vi "Replication and Deployment Utility.vi"() -> ()   [LabVIEW 2020]
uses:
  subVIs/TypeDefs/rad_State Data.ctl
  subVIs/Targets/TypeDefs/rad_Targets Settings.ctl
  subVIs/Targets/TypeDefs/rad_Target Information.ctl
  subVIs/Targets/TypeDefs/rad_Target Network Settings.ctl
  subVIs/App Images/TypeDefs/rad_App Images Settings.ctl
  subVIs/App Images/TypeDefs/rad_AppImage Information.ctl
  subVIs/App Images/TypeDefs/rad_Application Image Properties.ctl
  subVIs/App Images/TypeDefs/rad_FPGA Properties.ctl
  subVIs/App Images/TypeDefs/rad_FPGA Flash Properties.ctl
  subVIs/Targets/TypeDefs/rad_Discovery Settings.ctl
  subVIs/Util/Controls/Exit Button.ctl
  subVIs/Util/Controls/Retrieve Button.ctl
  subVIs/Util/Controls/Refresh Button.ctl
  subVIs/Util/Controls/Configure Button.ctl
  subVIs/Util/Controls/Deploy Button.ctl
  subVIs/Util/Controls/Select All Button.ctl
  subVIs/Util/Controls/Add Target Button.ctl
  subVIs/Util/Controls/Compare Button.ctl
  subVIs/Util/FP Control/FP Control Functions.ctl
  <vilib>/Utility/miscctls.llb/LVRowAndColumnUnsignedTypeDef.ctl
  subVIs/RT Image Compare/TypeDefs/rad_Comparison Modes.ctl
  <vilib>/nisyscfg/Close (System).vi
  subVIs/rad_Globals.vi
  <vilib>/nisyscfg/nisyscfg.lvlib
  <resource>/objmgr/nisysapi.rc
panel:
  in  "Targets Settings":bool
  in  "Refresh Targets":T1
  in  "Target List":i32[](listbox)=[0]
  in  "Add Target":T2
  in  "Select All":T3
  in  "Configure Targets":T4
  in  "Compare":T5
  in  "Deploy":T6
  in  "Retrieve":T7
  in  "State":T8 {"Targets Information"."Primary NIC"."IP Address Request Mode" items=["Static"=1, "DHCP/Link-Local"=2, "Link-Local Only"=4, "DHCP Only"=8]}
  in  "App Images Settings":bool
  in  "Refresh Apps":T1
  in  "Exit":T18
  in  "App Images List":i32(listbox)=6
  in  "Configure App":T4
  # "Deployment Targets"
  # "Application Images"
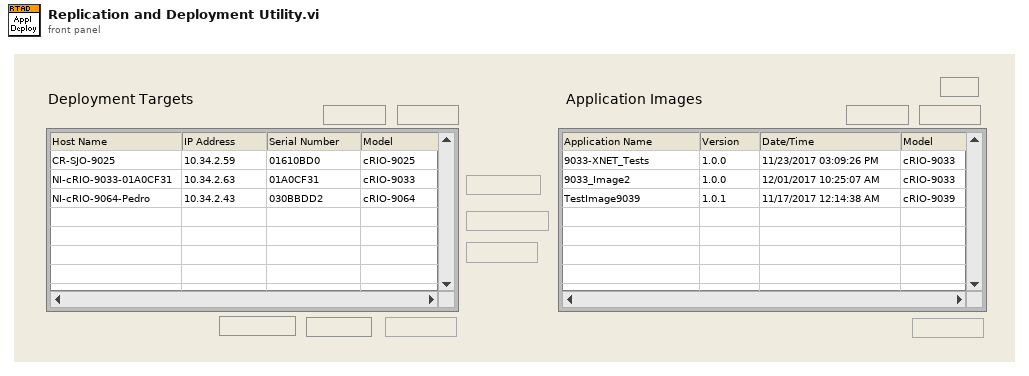
[diagram p1: front panel]
types:
  T1 = typedef "Refresh Button.ctl" = bool
  T2 = typedef "Add Target Button.ctl" = bool
  T3 = typedef "Select All Button.ctl" = bool
  T4 = typedef "Configure Button.ctl" = bool
  T5 = typedef "Compare Button.ctl" = bool
  T6 = typedef "Deploy Button.ctl" = bool
  T7 = typedef "Retrieve Button.ctl" = bool
  T8 = typedef "rad_State Data.ctl" = cluster{"Targets Settings":T9, "Targets Information":T10[], "App Images Settings":T12, "App Images Information":T13[], "Filtered Targets":i32[], "AppMode":string, "Configuration File Path":path, "Permissions":cluster{"Retrieve AppImgs":bool}, "User Added Targets":string[], "Discovery":T17}
  T9 = typedef "rad_Targets Settings.ctl" = cluster{"Target Types":string[], "Reduce Discovery Timeout":bool}
  T10 = typedef "rad_Target Information.ctl" = cluster{"Hostname":string, "Serial number":string, "Product name":string, "Product code":i32, "System status":string, "Credential type":enum16{"None/Unlocked", "FTP Password", "NIAuth Credentials"}, "User added?":bool, "Primary NIC":T11}
  T11 = typedef "rad_Target Network Settings.ctl" = cluster{"MAC address":string, "IP Address Request Mode":i32, "IP address":string, "Subnet mask":string, "Gateway":string, "DNS server":string}
  T12 = typedef "rad_App Images Settings.ctl" = cluster{"App Images Folder":path, "App Images Temp Folder":path, "CurrentVersion":string}
  T13 = typedef "rad_AppImage Information.ctl" = cluster{"AppImage Properties":T14, "AppImage Path":path}
  T14 = typedef "rad_Application Image Properties.ctl" = cluster{"Name":string, "Version":string, "Time":timestamp, "Description":string, "Key":string, "Chassis":string, "FPGA Properties":T15, "Model":string, "Retrieve":string[], "Deploy":string[], "Installed Software":string[]}
  T15 = typedef "rad_FPGA Properties.ctl" = T16[]
  T16 = typedef "rad_FPGA Flash Properties.ctl" = cluster{"Resource Name":string, "Path":path}
  T17 = typedef "rad_Discovery Settings.ctl" = cluster{"Method":u32, "NotAsk":bool, "IPsFilePath":path}
  T18 = typedef "Exit Button.ctl" = bool
  T19 = typedef "LVPoint32TypeDef.ctl" = cluster{"Horizontal":i32, "Vertical":i32}
  T20 = typedef "LVRowAndColumnTypeDef.ctl" = cluster{"Row":i32, "Column":i32}
  T21 = typedef "FP Control Functions.ctl" = enum16{"Open", "Close", "Bring To Front", "Center"}
  T22 = typedef "LVRowAndColumnUnsignedTypeDef.ctl" = cluster{"Row":u32, "Column":u32}
  T23 = typedef "rad_Comparison Modes.ctl" = enum32{"Compare Local Image With Controller", "Compare Two Local Images"}
  T24 = enum8{"Enabled", "Disabled", "Disabled and Grayed Out"}
  T25 = enum32{"invalid app kind", "Development System", "Run Time System", "Student Edition", "Embedded LabVIEW", "Evaluation", "Custom"}
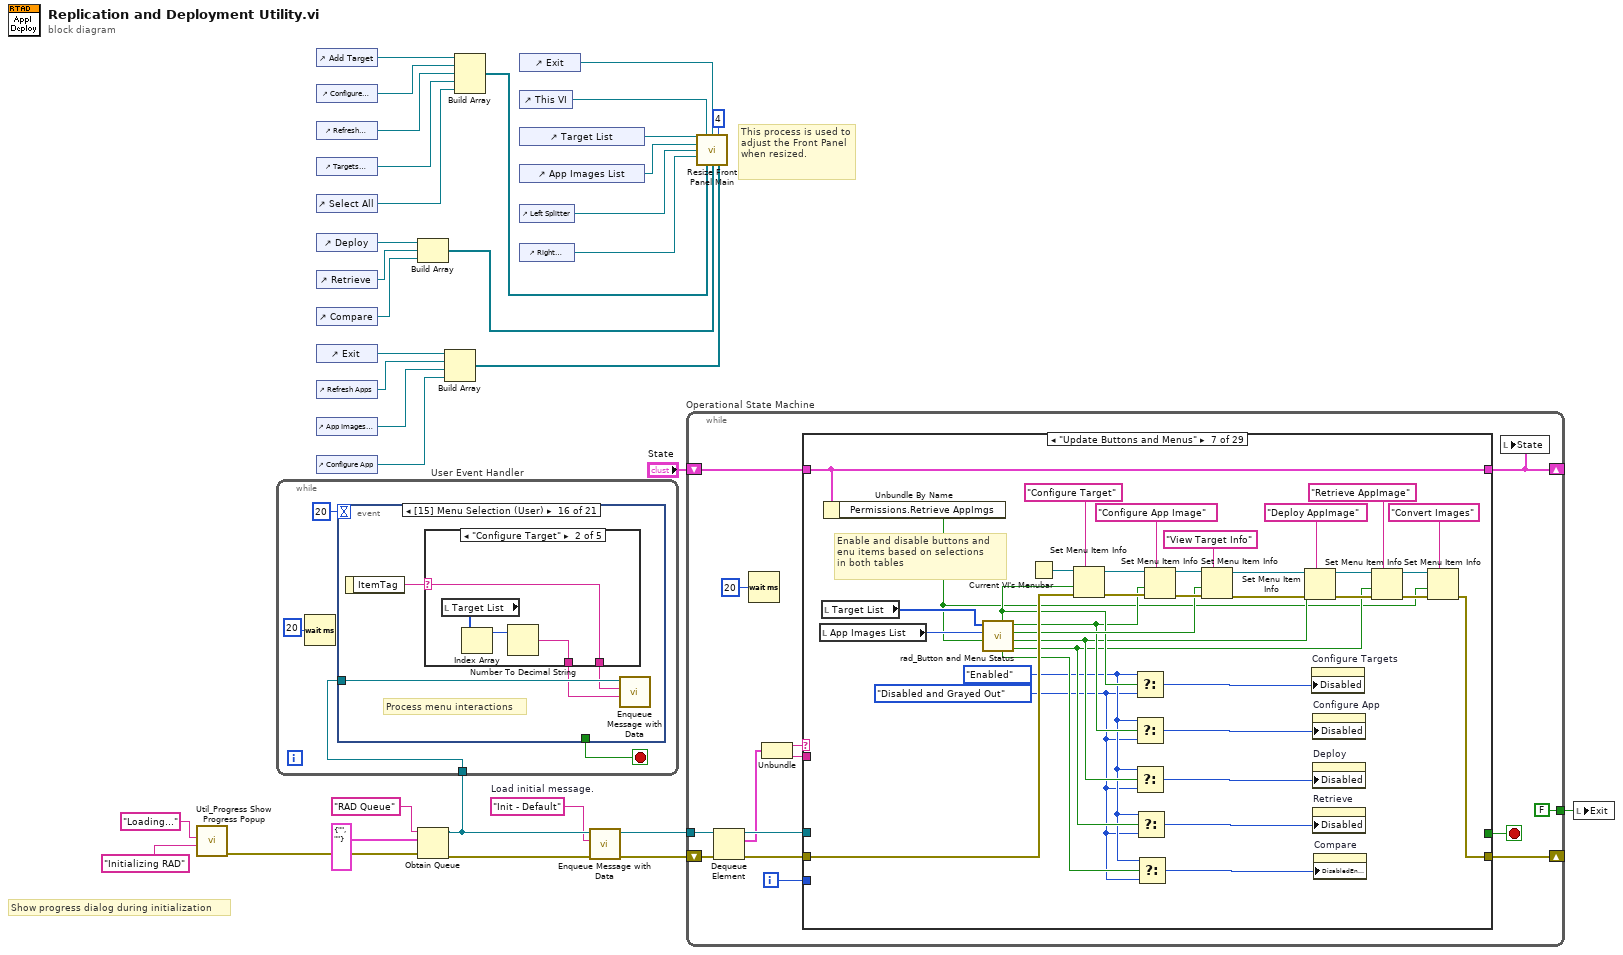
[diagram p0: block diagram]
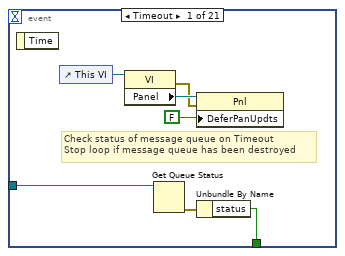
[diagram p2: hidden frame]
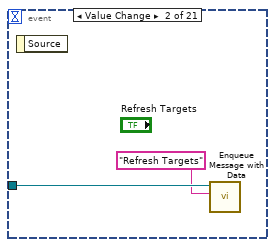
[diagram p3: hidden frame]
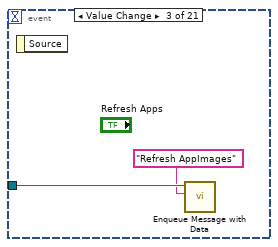
[diagram p4: hidden frame]
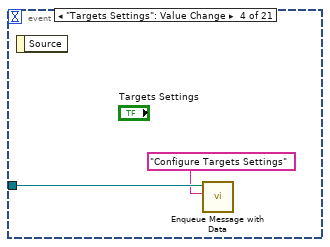
[diagram p5: hidden frame]
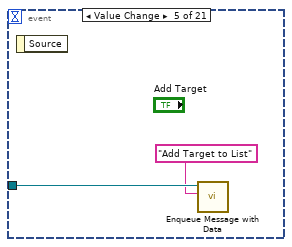
[diagram p6: hidden frame]
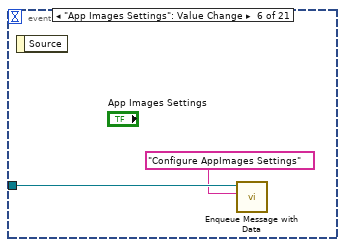
[diagram p7: hidden frame]
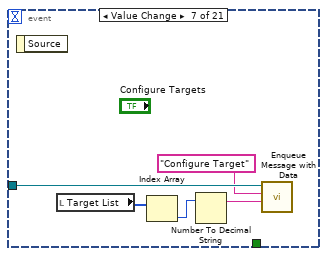
[diagram p8: hidden frame]
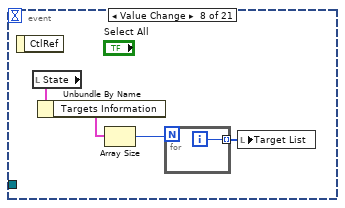
[diagram p9: hidden frame]
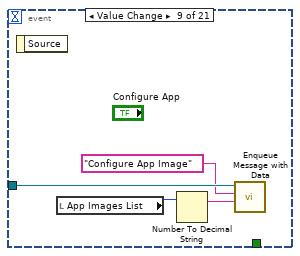
[diagram p10: hidden frame]
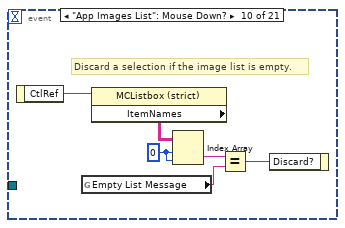
[diagram p11: hidden frame]
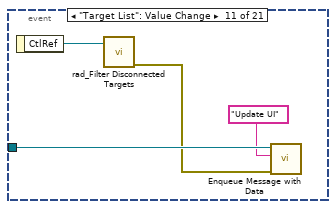
[diagram p12: hidden frame]
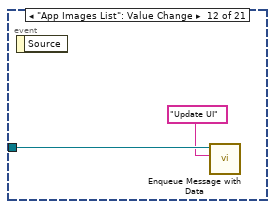
[diagram p13: hidden frame]
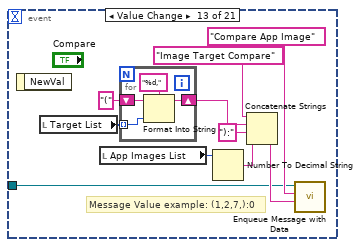
[diagram p14: hidden frame]
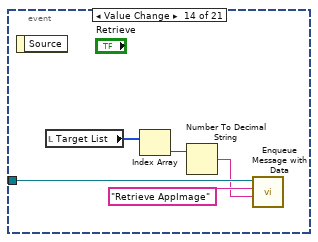
[diagram p15: hidden frame]
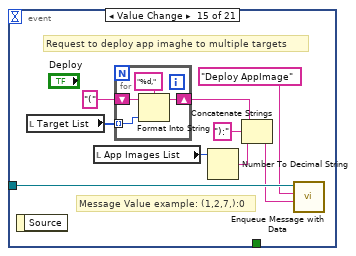
[diagram p16: hidden frame]
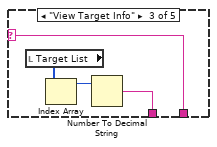
[diagram p18: hidden frame]
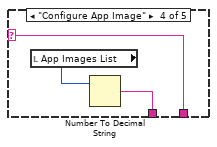
[diagram p19: hidden frame]
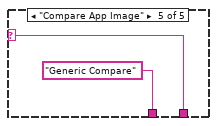
[diagram p20: hidden frame]
diagram:
  w4 = "Init - Default"  # Load initial message.
  # "Show progress dialog during initialization"
  # "This process is used to adjust the Front Panel when resized."
  n1 = call "Util_Progress Show Progress Popup.vi"("Title"="Initializing RAD", "Message"="Loading...") -> ("error out"=w1:errorcluster)  [unwired: 2 in, 7 out]
  n2 = control-ref of="Add Target"() -> (w25:refnum<vi>)
  n3 = control-ref of="Configure Targets"() -> (w24:refnum<vi>)
  n4 = control-ref of="Refresh Targets"() -> (w23:refnum<vi>)
  n5 = control-ref of="Targets Settings"() -> (w22:refnum<vi>)
  n6 = control-ref of="Select All"() -> (w21:refnum<vi>)
  n7 = control-ref of="Deploy"() -> (w19:refnum<vi>)
  n8 = control-ref of="Retrieve"() -> (w18:refnum<vi>)
  n9 = control-ref of="Compare"() -> (w17:refnum<vi>)
  n10 = control-ref of="Exit"() -> (w15:refnum<vi>)
  n11 = control-ref of="Refresh Apps"() -> (w14:refnum<vi>)
  n12 = control-ref of="App Images Settings"() -> (w13:refnum<vi>)
  n13 = control-ref of="Configure App"() -> (w12:refnum<vi>)
  n14 = Build Array(w19, w18, w17) -> (w16:refnum<vi>[])
  n15 = Obtain Queue(name (unnamed)="RAD Queue" ("message queue name"), element data type=cluster{string, string} {"", ""}, error in (no error)=w1) -> (queue out=w9:refnum<queue>, error out=w7:errorcluster)  [unwired: 2 in, 1 out]
  n16 = while "User Event Handler" {
    tunnel: w9 -> [w36]
    stop <- w37 stop-if-true
    n17 = Wait (ms)(milliseconds to wait=u32 20) -> ()  [unwired: 1 out]
    n18 = event shown="[15] Menu Selection (User)" {
      selector: _ -> [_ _ _ _ _ _ _ _ _ _ _ _ _ _ _ _ _ _ _ _ _]
      dyn-events: _ -> [_ _ _ _ _ _ _ _ _ _ _ _ _ _ _ _ _ _ _ _ _]
      timeout: 20 -> [_ _ _ _ _ _ _ _ _ _ _ _ _ _ _ _ _ _ _ _ _]
      tunnel: [w43 _ _ _ _ _ _ _ _ _ _ _ _ _ _ _ _ _ _ TRUE ("Discard?") w163] -> w37
      tunnel: w36 -> [w45 w47 w49 w51 w53 w55 w58 _ w68 _ w79 w81 w84 w98 w103 w116 w134 _ w153 w159 w162]
      event Timeout {
        # "Check status of message queue on Timeout\nStop loop if message queue has been destroyed"
        n19 = event-data() -> ()  [unwired: 2 out]
        n20 = control-ref of="This VI"() -> (w39:refnum<vi>)
        n21 = property class="VI"(reference=w39) -> (error out=w40:errorcluster, "Panel"=w42:refnum<vi>)  [unwired: 1 in, 1 out]
        n22 = Get Queue Status(queue=w45) -> (error out=w44:errorcluster)  [unwired: 1 in, 8 out]
        n23 = property class="Pnl"(reference=w42, error in=w40, "DeferPanUpdts"=FALSE ("Defer Panel Updates")) -> ()  [unwired: 2 out]
        n24 = Unbundle By Name(w44) -> ("status"=w43:bool)
      }
      event Value Change {
        n25 = event-data() -> ()  [unwired: 2 out]
        n26 = call "Enqueue Message with Data.vi"("message ID"="Refresh Targets", "queue in"=w47) -> ()  [unwired: 8 in, 2 out]
      }
      event Value Change {
        n27 = event-data() -> ()  [unwired: 2 out]
        n28 = call "Enqueue Message with Data.vi"("message ID"="Refresh AppImages", "queue in"=w49) -> ()  [unwired: 8 in, 2 out]
      }
      event "Targets Settings": Value Change {
        n29 = event-data() -> ()  [unwired: 2 out]
        n30 = call "Enqueue Message with Data.vi"("message ID"="Configure Targets Settings", "queue in"=w51) -> ()  [unwired: 8 in, 2 out]
      }
      event Value Change {
        n31 = event-data() -> ()  [unwired: 2 out]
        n32 = call "Enqueue Message with Data.vi"("message ID"="Add Target to List" ("Message Name"), "queue in"=w53) -> ()  [unwired: 8 in, 2 out]
      }
      event "App Images Settings": Value Change {
        n33 = event-data() -> ()  [unwired: 2 out]
        n34 = call "Enqueue Message with Data.vi"("message ID"="Configure AppImages Settings", "queue in"=w55) -> ()  [unwired: 8 in, 2 out]
      }
      event Value Change {
        n35 = event-data() -> ()  [unwired: 2 out]
        n36 = local read "Target List"() -> (w59:i32[])
        n37 = Index Array(array=w59) -> (element=w60:i32)  [unwired: 1 in]
        n38 = Number To Decimal String(number=w60) -> (decimal integer string=w56:string)  [unwired: 1 out]
        n39 = call "Enqueue Message with Data.vi"("extra data"=w56, "message ID"="Configure Target", "queue in"=w58) -> ()  [unwired: 7 in, 2 out]
      }
      event Value Change {
        n40 = event-data() -> ()  [unwired: 2 out]
        n41 = local read "State"() -> (w63:T8)
        n42 = Unbundle By Name(w63) -> ("Targets Information"=w62:T10[])
        n43 = Array Size(array=w62) -> (size(s)=w61:i32)
        n44 = for {
          N: w61 -> [_]
          tunnel: [w65] -> w64 mode=indexing
          i -> [w65]
        }
        n45 = local write "Target List"(w64) -> ()
      }
      event Value Change {
        n46 = event-data() -> ()  [unwired: 2 out]
        n47 = local read "App Images List"() -> (w69:i32)
        n48 = Number To Decimal String(number=w69) -> (decimal integer string=w66:string)  [unwired: 1 out]
        n49 = call "Enqueue Message with Data.vi"("extra data"=w66, "message ID"="Configure App Image", "queue in"=w68) -> ()  [unwired: 7 in, 2 out]
      }
      event "App Images List": Mouse Down? {
        w73 = 0 ("index (row)")
        # "Discard a selection if the image list is empty."
        n50 = event-data() -> ("CtlRef"=w75:refnum<vi>)  [unwired: 1 out]
        n51 = global read "rad_Globals.vi" "Empty List Message"() -> (w71:string)
        n52 = property class="MCListbox (strict)"(reference=w75) -> ("ItemNames"=w74:string[][])  [unwired: 1 in, 2 out]
        n53 = Index Array(array=w74, index (row)=w73, index (col)=w73) -> (element=w72:string)
        n54 = Equal?(x=w72, y=w71) -> (x = y?=w70:bool)
        n55 = event-data("Discard?"=w70) -> ()  [unwired: 1 in, 1 out]
      }
      event "Target List": Value Change {
        n56 = event-data() -> ("CtlRef"=w77:refnum<vi>)  [unwired: 1 out]
        n57 = call "rad_Filter Disconnected Targets.vi"("Target List Ref"=w77) -> ("error out"=w76:errorcluster)  [unwired: 10 in]
        n58 = call "Enqueue Message with Data.vi"("error in (no error)"=w76, "message ID"="Update UI" ("Message"), "queue in"=w79) -> ()  [unwired: 7 in, 2 out]
      }
      event "App Images List": Value Change {
        n59 = event-data() -> ()  [unwired: 2 out]
        n60 = call "Enqueue Message with Data.vi"("message ID"="Update UI" ("Message"), "queue in"=w81) -> ()  [unwired: 8 in, 2 out]
      }
      event Value Change {
        # "Message Value example: (1,2,7,):0"
        n61 = event-data() -> ()  [unwired: 2 out]
        n62 = local read "Target List"() -> (w88:i32[])
        n63 = local read "App Images List"() -> (w87:i32)
        n64 = for {
          shift-right: [w95] -> w89
          shift-left: "(" -> [w93]
          tunnel: w88 -> [w94] mode=indexing
          n65 = Format Into String(format string="%d,", initial string=w93, w94) -> (resulting string=w95:string)  [unwired: 1 in, 1 out]
        }
        n66 = Number To Decimal String(number=w87) -> (decimal integer string=w86:string)  [unwired: 1 out]
        n67 = Concatenate Strings("Image Target Compare" ("string"), w89, "):" ("string"), w86) -> (w91:string)
        n68 = call "Enqueue Message with Data.vi"("extra data"=w91, "message ID"="Compare App Image", "queue in"=w84) -> ()  [unwired: 7 in, 2 out]
      }
      event Value Change {
        n69 = event-data() -> ()  [unwired: 2 out]
        n70 = local read "Target List"() -> (w99:i32[])
        n71 = Index Array(array=w99) -> (element=w100:i32)  [unwired: 1 in]
        n72 = Number To Decimal String(number=w100) -> (decimal integer string=w96:string)  [unwired: 1 out]
        n73 = call "Enqueue Message with Data.vi"("extra data"=w96, "message ID"="Retrieve AppImage", "queue in"=w98) -> ()  [unwired: 7 in, 2 out]
      }
      event Value Change {
        # "Request to deploy app imaghe to multiple targets"
        # "Message Value example: (1,2,7,):0"
        n74 = event-data() -> ()  [unwired: 2 out]
        n75 = local read "Target List"() -> (w105:i32[])
        n76 = local read "App Images List"() -> (w107:i32)
        n77 = for {
          shift-right: [w113] -> w104
          shift-left: "(" -> [w111]
          tunnel: w105 -> [w112] mode=indexing
          n78 = Format Into String(format string="%d,", initial string=w111, w112) -> (resulting string=w113:string)  [unwired: 1 in, 1 out]
        }
        n79 = Number To Decimal String(number=w107) -> (decimal integer string=w108:string)  [unwired: 1 out]
        n80 = Concatenate Strings(w104, "):" ("string"), w108) -> (w101:string)
        n81 = call "Enqueue Message with Data.vi"("extra data"=w101, "message ID"="Deploy AppImage", "queue in"=w103) -> ()  [unwired: 7 in, 2 out]
      }
      event Menu Selection (User) {
        # "Process menu interactions"
        n82 = event-data() -> ("ItemTag"=w117:string)  [unwired: 1 out]
        n83 = case shown="\"Configure Target\"" w117 {
          selector: w117 -> [w118 w120 w124 w128 w130]
          tunnel: [w118 w120 w124 w128 w130] -> w115
          tunnel: [_ w119 w123 w127 "Generic Compare"] -> w114
          frame Default {
          }
          frame "Configure Target" {
            n84 = local read "Target List"() -> (w122:i32[])
            n85 = Index Array(array=w122) -> (element=w121:i32)  [unwired: 1 in]
            n86 = Number To Decimal String(number=w121) -> (decimal integer string=w119:string)  [unwired: 1 out]
          }
          frame "View Target Info" {
            n87 = local read "Target List"() -> (w126:i32[])
            n88 = Index Array(array=w126) -> (element=w125:i32)  [unwired: 1 in]
            n89 = Number To Decimal String(number=w125) -> (decimal integer string=w123:string)  [unwired: 1 out]
          }
          frame "Configure App Image" {
            n90 = local read "App Images List"() -> (w129:i32)
            n91 = Number To Decimal String(number=w129) -> (decimal integer string=w127:string)  [unwired: 1 out]
          }
          frame "Compare App Image" {
          }
        }
        n92 = call "Enqueue Message with Data.vi"("extra data"=w114, "message ID"=w115, "queue in"=w116) -> ()  [unwired: 7 in, 2 out]
      }
      event "Target List": Shortcut Menu Selection (User) {
        n93 = event-data() -> ("CtlRef"=w136:refnum<vi>, "Coords"=w135:T19, "ItemTag"=w133:string)  [unwired: 2 out]
        n94 = invoke class="MCListbox (strict)" method="Point To Row Column"(reference=w136, "Point"=w135) -> ("CellPosition"=w138:T20)  [unwired: 5 in, 6 out]
        n95 = Unbundle By Name(w138) -> ("Row"=w137:i32)
        n96 = Number To Decimal String(number=w137) -> (decimal integer string=w132:string)  [unwired: 1 out]
        n97 = call "Enqueue Message with Data.vi"("extra data"=w132, "message ID"=w133, "queue in"=w134) -> ()  [unwired: 7 in, 2 out]
      }
      event "App Images List": Shortcut Menu Activation? {
        n98 = event-data() -> ("MenuRef"=w140:refnum<k9>)  [unwired: 1 out]
        n99 = global read "rad_Globals.vi" "Manager Permissions"() -> (w139:bool)
        n100 = case shown="False" w139 {
          tunnel: w140 -> [w145 _]
          tunnel: [w142 _] -> _
          frame False {
            w141 = string[] ["View App Image Info"] ("item names")
            n101 = Delete Menu Items(9:w145) -> (0:w143:errorcluster, 3:w144:refnum<k9>)  [unwired: 3 in]
            n102 = Insert Menu Items(6:w143, 7:w141, 8:w141, 9:w144) -> (0:w142:errorcluster)  [unwired: 2 in, 2 out]
          }
          frame True {
          }
        }
        n103 = event-data() -> ()  [unwired: 2 in, 1 out]
      }
      event "App Images List": Shortcut Menu Selection (User) {
        n104 = event-data() -> ("CtlRef"=w155:refnum<vi>, "Coords"=w154:T19, "ItemTag"=w146:string)  [unwired: 1 out]
        n105 = Equal?(x=w146, y="Compare App Image") -> (x = y?=w151:bool)
        n106 = invoke class="MCListbox (strict)" method="Point To Row Column"(reference=w155, "Point"=w154) -> ("CellPosition"=w157:T20)  [unwired: 5 in, 6 out]
        n107 = Unbundle By Name(w157) -> ("Row"=w156:i32)
        n108 = Number To Decimal String(number=w156) -> (decimal integer string=w148:string)  [unwired: 1 out]
        n109 = Concatenate Strings("Only Image Selected(" ("string"), w148) -> (w150:string)
        n110 = Select(t=w150, s=w151, f=w148) -> (s? t:f=w147:string)
        n111 = call "Enqueue Message with Data.vi"("extra data"=w147, "message ID"=w146, "queue in"=w153) -> ()  [unwired: 7 in, 2 out]
      }
      event Value Change {
        n112 = event-data() -> ()  [unwired: 2 out]
        n113 = call "Enqueue Message with Data.vi"("message ID"="Exit", "queue in"=w159) -> ()  [unwired: 8 in, 2 out]
      }
      event Panel Close? {
        w163 = TRUE ("Discard?")
        # "Intercepts the upper right close panel\noperation to allow a smooth shutdown\nas opposed to immediately killing the app."
        n114 = event-data() -> ()  [unwired: 2 out]
        n115 = call "Enqueue Message with Data.vi"("message ID"="Exit", "queue in"=w162) -> ()  [unwired: 8 in, 2 out]
        n116 = event-data("Discard?"=w163) -> ()  [unwired: 1 in, 1 out]
      }
    }
  }
  n117 = Build Array(w15, w14, w13, w12) -> (w11:refnum<vi>[])
  n118 = Build Array(w25, w24, w23, w22, w21) -> (w20:refnum<vi>[])
  n119 = control-ref of="Exit"() -> (w31:refnum<vi>)
  n120 = control-ref of="This VI"() -> (w30:refnum<vi>)
  n121 = control-ref of="Target List"() -> (w29:refnum<vi>)
  n122 = control-ref of="App Images List"() -> (w28:refnum<vi>)
  n123 = control-ref of="Left Splitter"() -> (w27:refnum<vi>)
  n124 = control-ref of="Right Splitter"() -> (w26:refnum<vi>)
  n125 = call "Enqueue Message with Data.vi"("error in (no error)"=w7, "message ID"=w4, "queue in"=w9) -> ("error out"=w6:errorcluster, "queue out"=w8:refnum<queue>)  [unwired: 7 in]
  n126 = while "Operational State Machine" {
    shift-left: w6 -> [w169]
    shift-right: [w170] -> _
    tunnel: w8 -> [w174]
    shift-left: "State" -> [w177]
    shift-right: [w171] -> _
    tunnel: [T18 FALSE ("Exit")] -> w10
    i -> [w173]
    stop <- w167 stop-if-true
    n127 = Dequeue Element(queue=w174, error in (no error)=w169) -> (queue out=w176:refnum<queue>, element=w172:cluster{string, string}, error out=w175:errorcluster)  [unwired: 1 in, 1 out]
    n128 = Wait (ms)(milliseconds to wait=u32 20) -> ()  [unwired: 1 out]
    n129 = Unbundle(w172) -> (w166:string, w165:string)
    n130 = case shown="\"Update Buttons and Menus\"" w166 {
      tunnel: [w179 w181 w195 w223 w245 w266 w297 w312 w314 w318 w324 w336 w348 w366 w382 w404 w420 w436 w449 w460 w462 w483 w498 w510 w518 w587 w602 w634 w650] -> w171
      tunnel: w177 -> [w179 w181 w199 w222 w246 w262 w297 w312 w314 w318 w324 w336 w342 w367 w383 w405 w421 w436 w454 w460 w466 w484 w497 w510 w518 w587 w603 w634 w650]
      tunnel: w176 -> [_ _ w183 w206 _ w258 _ _ _ _ w331 _ w346 w364 w378 w403 w419 _ w448 _ w464 w477 w500 _ _ w574 w606 w619 w651]
      tunnel: w175 -> [w178 w180 w188 w205 w244 w260 w294 w313 w315 w317 w330 w335 w345 w363 w380 w399 w418 w429 w447 w459 w463 w479 w499 w511 w517 w576 w609 w622 w655]
      tunnel: w173 -> [_ _ _ _ _ _ _ _ _ _ _ _ _ _ _ _ _ _ _ _ _ _ _ _ _ _ _ _ _]
      tunnel: w165 -> [_ _ _ _ _ _ _ _ _ _ _ _ w339 _ _ w413 _ w434 w458 _ _ w487 _ w507 w514 w585 w611 w633 _]
      tunnel: [w178 w180 w182 w207 w244 w259 w278 w313 w315 errorcluster {"status"=FALSE, "code"=0, "source"=""} ("error out") w325 w335 w347 w365 w379 w401 w415 w429 w446 w459 w465 w478 w494 w511 w512 w575 w607 w621 w652] -> w170
      tunnel: [_ _ _ _ _ _ _ _ _ _ TRUE _ _ _ _ _ _ _ _ _ _ _ _ _ _ _ _ _ _] -> w167
      frame "Missing Message Handler", Default {
      }
      frame "**** General Application Messages ****" {
      }
      frame "Init - Default" {
        w189 = T22 {"Row"=0, "Column"=0} ("Top Left Visible Cell")
        w191 = string[][] [] ("Item Names")
        w198 = u8 2 ("Disabled")
        # "Initialize the UI"
        # "Application Folder"
        # "Default AppImages folder"
        n131 = call "Util_App Application Directory.vi"() -> ("Application Directory"=w194:path)  [unwired: 11 out]
        n132 = call "Enqueue Message with Data.vi"("error in (no error)"=w188, "message ID"="Init - Load Config", "queue in"=w183) -> ("error out"=w187:errorcluster, "queue out"=w186:refnum<queue>)  [unwired: 7 in]
        n133 = local write "App Images List"(-1 ("App Images List")) -> ()
        n134 = local write "Target List"(i32[] [] ("Target List")) -> ()
        n135 = Build Path(base path=w194, name or relative path="appimages") -> (appended path=w200:path)
        n136 = Build Path(base path=w194, name or relative path="rad_config.ini" ("Config File Name")) -> (appended path=w192:path)
        n137 = call "Enqueue Message with Data.vi"("error in (no error)"=w187, "message ID"="Init - Configure Settings", "queue in"=w186) -> ("error out"=w182:errorcluster)  [unwired: 7 in, 1 out]
        n138 = property on="Configure App" class="Bool"("Disabled"=w198) -> ()  [unwired: 2 in, 2 out]
        n139 = property on="Configure Targets" class="Bool"("Disabled"=w198) -> ()  [unwired: 2 in, 2 out]
        n140 = Bundle By Name(cluster=w199, "App Images Settings.App Images Folder"=w200, "Configuration File Path"=w192) -> (w195:T8)
        n141 = property on="Target List" class="MCListbox (strict)"("ItemNames"=w191, "TopLeft"=w189) -> ()  [unwired: 2 in, 2 out]
        n142 = property on="App Images List" class="MCListbox (strict)"("ItemNames"=w191, "TopLeft"=w189) -> ()  [unwired: 2 in, 2 out]
        n143 = call "Util_FP Control.vi"("Function"=FP_Control_Functions."Center") -> ()  [unwired: 10 in, 1 out]
      }
      frame "Init - Load Config" {
        # "Close Init\nDialog"
        n144 = call "rad_Load Config.vi"("error in (no error"=w205, "State in"=w222) -> ("error out"=w203:errorcluster, "State out"=w223:T8)  [unwired: 1 in, 7 out]
        n145 = call <vilib>:"Initialize Session.vi"("error in (no error)"=w203) -> ("error out"=w210:errorcluster, "Session out"=w211:refnum<k21>)  [unwired: 9 in]
        n146 = property class="System Session"(reference=w211, error in=w210) -> (reference out=w212:refnum<k21>, error out=w209:errorcluster, "InstalledVer"=w208:string)
        n147 = Scan From String(format string="%d.%d.%d", input string=w208) -> (output 1=w220:i32, output 2=w217:i32, output 3=w214:i32)  [unwired: 5 in, 3 out]
        n148 = call-poly <vilib>:"Close.vi"("error in (no error)"=w209, "Session in"=w212) -> ("error out"=w202:errorcluster)  [unwired: 9 in]
        n149 = Multiply(x=10, y=w217) -> (x*y=w215:i32)
        n150 = Multiply(x=100, y=w220) -> (x*y=w216:i32)
        n151 = call "Util_Progress Close Progress Popup.vi"("error in (no error)"=w202) -> ()  [unwired: 2 in, 9 out]
        n152 = Compound Arithmetic op=ADD(w216, w215, w214) -> (w213:i32)
        n153 = case shown="Default" w213 {
          tunnel: [w235 TRUE ("T button?")] -> w204
          frame Default {
            n154 = Two Button Dialog(message="RAD requires newer functionality\nthan the software you have installed.\nPlease update to NI System Configuration\nversion 14.0 or higher.", 1:"Exit" ("F button name (\"Cancel\")"), 2:"Continue" ("T button name (\"OK\")")) -> (T button?=w235:bool)
          }
          frame 1400.. {
            # "RAD 14.0 has been fully tested\nwith NI System Configuration 14.0.\nFuture versions should work fine too."
          }
        }
        n155 = case shown="True" w204 {
          tunnel: w203 -> [w225 w233]
          tunnel: [w226 w228] -> w207
          tunnel: w206 -> [_ w232]
          frame False {
            n156 = property on="Exit" class="Bool (strict)"(error in=w225, "Val(Sgnl)"=T18 TRUE ("Value (Signaling)")) -> (error out=w226:errorcluster)  [unwired: 1 in, 1 out]
          }
          frame True {
            n157 = call "Enqueue Message with Data.vi"("error in (no error)"=w233, "extra data"="First", "message ID"="Configure Discovery", "queue in"=w232) -> ("error out"=w229:errorcluster, "queue out"=w230:refnum<queue>)  [unwired: 6 in]
            n158 = call "Enqueue Message with Data.vi"("error in (no error)"=w229, "message ID"="Refresh AppImages", "queue in"=w230) -> ("error out"=w228:errorcluster)  [unwired: 7 in, 1 out]
          }
        }
      }
      frame "Init - Configure Settings" {
        # "The temp folder should always be writable."
        # "Set permissions and update UI based on application\nmode. Disable or hide controls not appropriate\nfor current application mode."
        # "Apply configuration settings from config file"
        n159 = Unbundle By Name(w246) -> ("AppMode"=w247:string)
        n160 = case shown="\"Manager\"" w247 {
          tunnel: [TRUE ("Visible") FALSE ("Visible")] -> w243
          frame "Manager" {
          }
          frame Default {
          }
        }
        n161 = call <vilib>:"Generate Temporary File Path.vi"("Temporary File Extension (tmp)"="rad") -> ("Unique Temporary File Path"=w240:path)  [unwired: 9 in, 1 out]
        n162 = property on="Retrieve" class="Bool"("Visible"=w243) -> ()  [unwired: 2 in, 2 out]
        n163 = property on="Configure App" class="Bool"("Visible"=w243) -> ()  [unwired: 2 in, 2 out]
        n164 = Bundle By Name(cluster=w246, "App Images Settings.App Images Temp Folder"=w240, "Permissions.Retrieve AppImgs"=w243) -> (w245:T8)
        n165 = global write "rad_Globals.vi" "Manager Permissions"(w243) -> ()
        n166 = global write "rad_Globals.vi" "ShownImageVersionDialog"(FALSE ("ShownNewerVersionDialog")) -> ()
      }
      frame "Update UI" {
        # "Scroll the lists to the top if no item is selected."
        # "Display target and app images based on settings\nfor each of these tables"
        n167 = Unbundle By Name(w262) -> ("Targets Information"=w269:T10[], "Targets Settings.Target Types"=w261:string[], "App Images Information"=w263:T13[])
        n168 = call "rad_Format Application Images Information.vi"("App Images Information"=w263) -> ("App Images Information"=w264:string[][])  [unwired: 10 out]
        n169 = call "rad_FilterTargets.vi"("Target Types"=w261, "Targets Information"=w269) -> ("Filtered Targets"=w267:i32[], "Targets Information"=w268:T10[])  [unwired: 8 out]
        n170 = Bundle By Name(cluster=w262, "Filtered Targets"=w267) -> (w266:T8)
        n171 = call "rad_Format Target Information.vi"("Targets Information"=w268) -> ("Targets Information"=w265:string[][])  [unwired: 10 out]
        n172 = property on="App Images List" class="MCListbox (strict)"("ItemNames"=w264) -> (error out=w255:errorcluster)  [unwired: 2 in, 1 out]
        n173 = property on="Target List" class="MCListbox (strict)"("ItemNames"=w265) -> (error out=w256:errorcluster)  [unwired: 2 in, 1 out]
        n174 = flat-sequence {
          tunnel: w256 -> [_]
          tunnel: w255 -> [_]
          tunnel: ["App Images List"] -> w253
          tunnel: [w273] -> w254
          tunnel: [-1 ("y")] -> w251
          frame #0 {
            n175 = Array Size(array="Target List") -> (size(s)=w273:i32)
          }
        }
        n176 = Equal?(x=w253, y=w251) -> (x = y?=w250:bool)
        n177 = Equal To 0?(x=w254) -> (x = 0?=w252:bool)
        n178 = call "Enqueue Message with Data.vi"("error in (no error)"=w260, "message ID"="Update Buttons and Menus" ("Message Name"), "queue in"=w258) -> ("error out"=w259:errorcluster)  [unwired: 7 in, 1 out]
        n179 = case shown="True" w250 {
          frame False {
          }
          frame True {
            n180 = property on="App Images List" class="MCListbox (strict)"("TopLeft"=T22 {"Row"=0, "Column"=0} ("Top Left Visible Cell")) -> ()  [unwired: 2 in, 2 out]
          }
        }
        n181 = case shown="True" w252 {
          frame False {
          }
          frame True {
            n182 = property on="Target List" class="MCListbox (strict)"("TopLeft"=T22 {"Row"=0, "Column"=0} ("Top Left Visible Cell")) -> ()  [unwired: 2 in, 2 out]
          }
        }
      }
      frame "Update Buttons and Menus" {
        w282 = T24."Disabled and Grayed Out" ("Disabled")
        w283 = T24."Enabled" ("Disabled")
        # "Enable and disable buttons and \nenu items based on selections\nin both tables"
        n183 = local read "App Images List"() -> (w295:i32)
        n184 = local read "Target List"() -> (w296:i32[])
        n185 = Unbundle By Name(w297) -> ("Permissions.Retrieve AppImgs"=w276:bool)
        n186 = call "rad_Button and Menu Status.vi"("Manager Permissions"=w276, "App Image List"=w295, "Target List"=w296) -> ("Retrieve AppImage"=w286:bool, "Deploy AppImage"=w288:bool, "View Target Info"=w293:bool, "Configure App Image"=w290:bool, "Compare"=w284:bool, "Configure Target"=w292:bool)  [unwired: 3 in]
        n187 = Current VI's Menubar() -> (w298:refnum<k9>)
        n188 = Set Menu Item Info(7:"Configure Target" ("item tag"), 8:w294, 9:w292, 11:w298) -> (0:w300:errorcluster, 3:w302:refnum<k9>)  [unwired: 3 out]
        n189 = Select(t=w283, s=w292, f=w282) -> (s? t:f=w291:T24)
        n190 = Select(t=w283, s=w290, f=w282) -> (s? t:f=w289:T24)
        n191 = Select(t=w283, s=w288, f=w282) -> (s? t:f=w287:T24)
        n192 = Select(t=w283, s=w286, f=w282) -> (s? t:f=w285:T24)
        n193 = Select(t=w283, s=w284, f=w282) -> (s? t:f=w281:T24)
        n194 = Set Menu Item Info(7:"Configure App Image" ("item tag"), 8:w300, 9:w290, 11:w302) -> (0:w303:errorcluster, 3:w304:refnum<k9>)  [unwired: 3 out]
        n195 = Set Menu Item Info(7:"View Target Info" ("item tag"), 8:w303, 9:w293, 11:w304) -> (0:w305:errorcluster, 3:w306:refnum<k9>)  [unwired: 3 out]
        n196 = Set Menu Item Info(7:"Deploy AppImage" ("item tag"), 8:w305, 9:w288, 11:w306) -> (0:w307:errorcluster, 3:w308:refnum<k9>)  [unwired: 3 out]
        n197 = property on="Configure Targets" class="Bool"("Disabled"=w291) -> ()  [unwired: 2 in, 2 out]
        n198 = property on="Configure App" class="Bool"("Disabled"=w289) -> ()  [unwired: 2 in, 2 out]
        n199 = property on="Deploy" class="Bool"("Disabled"=w287) -> ()  [unwired: 2 in, 2 out]
        n200 = property on="Retrieve" class="Bool"("Disabled"=w285) -> ()  [unwired: 2 in, 2 out]
        n201 = property on="Compare" class="Bool"("DisabledEnum"=w281) -> ()  [unwired: 2 in, 2 out]
        n202 = Set Menu Item Info(7:"Retrieve AppImage" ("item tag"), 8:w307, 9:w286, 11:w308) -> (0:w279:errorcluster, 3:w280:refnum<k9>)  [unwired: 3 out]
        n203 = Set Menu Item Info(7:"Convert Images" ("item tag"), 8:w279, 9:w276, 11:w280) -> (0:w278:errorcluster)  [unwired: 4 out]
      }
      frame "Status" {
      }
      frame "About" {
        # "Show About dialog"
        n204 = call "rad_About Dialog.vi"() -> ()  [unwired: 12 out]
      }
      frame "Error" {
        # "Display run-time error message\nAdd code to log error if desired"
        n205 = disable-structure shown="TARGET_TYPE==Windows" {
          disable-tunnel: w317 -> [w319 _]
          frame condition #0 (active) {
            n206 = call <vilib>:"Simple Error Handler.vi"("error in (no error)"=w319) -> ()  [unwired: 1 in, 8 out]
          }
          frame condition #1 {
          }
        }
      }
      frame "Exit" {
        # "Store current settings in the application config file"
        # "Close the front panel if the application is running as an EXE"
        n207 = Release Queue(queue=w331, force destroy? (F)=TRUE, error in (no error)=w330) -> (error out=w323:errorcluster)  [unwired: 2 out]
        n208 = Open Application Reference() -> (0:w328:errorcluster, 3:w329:refnum<vi>)  [unwired: 4 in]
        n209 = call "rad_Save Config.vi"("error in (no error"=w323, "State"=w324) -> ("error out"=w322:errorcluster)  [unwired: 1 in, 8 out]
        n210 = property class="App"(reference=w329, error in=w328) -> ("App.Kind"=w327:T25)  [unwired: 2 out]
        n211 = case shown="\"Run Time System\"" w327 {
          frame Default {
          }
          frame "Run Time System" {
            # "Close FP in EXE"
            n212 = Current VI's Path() -> (path=w334:path)
            n213 = Open VI Reference(vi path=w334) -> (vi reference=w333:refnum<vi>, error out=w332:errorcluster)  [unwired: 5 in]
            n214 = invoke class="VI" method="FP.Close"(reference=w333, error in=w332) -> ()  [unwired: 1 in, 3 out]
          }
        }
        n215 = property on="Exit" class="Bool (strict)"(error in=w322, "Val(Sgnl)"=TRUE) -> (error out=w325:errorcluster)  [unwired: 1 in, 1 out]
      }
      frame "**** Target Messages ****" {
      }
      frame "Configure Discovery" {
        # "Refresh targets if:\n-It is the first iteration OR\n-Discovery settings were just changed"
        # "We ask the user to select the discovery \nmethod only if:\n-It is being called from the top\nmenu (not first) OR\n-The NotAsk flag hasn't been set to \nTrue (still ask me) in a first call"
        n216 = Unbundle By Name(w342) -> ("Discovery.NotAsk"=w341:bool)
        n217 = Equal?(x=w339, y="First") -> (x = y?=w337:bool)
        n218 = Compound Arithmetic op=OR(invert w341, invert w337) -> (w340:bool)
        n219 = case shown="True" w340 {
          tunnel: w342 -> [w355 w358]
          tunnel: [w355 w357] -> w348
          tunnel: [FALSE ("Changes?") w356] -> w343
          frame False {
          }
          frame True {
            # "This VI will ask the user\nhow to discover targets\non the network"
            n220 = call "rad_Configure Discovery Settings Dialog.vi"("Discovery Settings"=w358) -> ("Changes?"=w356:bool, "Discovery Settings out"=w357:T8)  [unwired: 9 in]
          }
        }
        n221 = Or(x=w343, y=w337) -> (x .or. y?=w344:bool)
        n222 = case shown="False" w344 {
          tunnel: [w349 w352] -> w347
          tunnel: w346 -> [_ w351]
          tunnel: w345 -> [w349 w350]
          frame False {
          }
          frame True {
            n223 = call "Enqueue Message with Data.vi"("error in (no error)"=w350, "message ID"="Refresh Targets" ("Message Name"), "queue in"=w351) -> ("error out"=w352:errorcluster)  [unwired: 7 in, 1 out]
          }
        }
      }
      frame "Refresh Targets" {
        # "Refresh list of RT targets on the local subnet.\nShow progress dialog during this process."
        n224 = Unbundle By Name(w367) -> ("Targets Settings.Reduce Discovery Timeout"=w360:bool, "User Added Targets"=w373:string[], "Targets Settings.Target Types"=w359:string[])
        n225 = call "Util_Progress Show Progress Popup.vi"("error in (no error)"=w363, "Title"="Discovering Targets", "Message"="Refreshing target list...") -> ("error out"=w361:errorcluster)  [unwired: 1 in, 7 out]
        n226 = Search 1D Array(1D array=w359, element="User Targets Only") -> (index of element=w370:i32)  [unwired: 1 in]
        n227 = Not Equal?(x=w370, y=-1) -> (x != y?=w368:bool)
        n228 = call "rad_Refresh Target Information.vi"("Reduce Discovery Timeout"=w360, "error in (no error)"=w361, "User Added Targets Only"=w368, "User Added Targets"=w373) -> ("error out"=w362:errorcluster, "Targets Information"=w372:T10[])  [unwired: 6 in]
        n229 = call "Util_Progress Close Progress Popup.vi"("error in (no error)"=w362) -> ()  [unwired: 2 in, 9 out]
        n230 = Bundle By Name(cluster=w367, "Targets Information"=w372) -> (w366:T8)
        n231 = call "Enqueue Message with Data.vi"("error in (no error)"=w362, "message ID"="Update UI", "queue in"=w364) -> ("error out"=w365:errorcluster)  [unwired: 7 in, 1 out]
      }
      frame "Add Target to List" {
        n232 = Unbundle By Name(w383) -> ("User Added Targets"=w385:string[])
        n233 = call "rad_Add Target By IP Dialog.vi"() -> ("Canceled?"=w377:bool, "IP Address"=w384:string)  [unwired: 10 in]
        n234 = case shown="False" w377 {
          tunnel: w385 -> [w393 w398]
          tunnel: w384 -> [w392 _]
          tunnel: [w394 w398] -> w381
          frame False {
            n235 = Search 1D Array(1D array=w393, element=w392) -> (index of element=w397:i32)  [unwired: 1 in]
            n236 = Build Array (concatenate)(w393, w392) -> (w391:string[])
            n237 = Not Equal?(x=w397, y=-1) -> (x != y?=w395:bool)
            n238 = Select(t=w393, s=w395, f=w391) -> (s? t:f=w394:string[])
          }
          frame True {
          }
        }
        n239 = case shown="False" w377 {
          tunnel: w380 -> [w389 w390]
          tunnel: [w388 w390] -> w379
          tunnel: w378 -> [w387 _]
          frame False {
            n240 = call "Enqueue Message with Data.vi"("error in (no error)"=w389, "message ID"="Refresh Targets" ("Message Name"), "queue in"=w387) -> ("error out"=w388:errorcluster)  [unwired: 7 in, 1 out]
          }
          frame True {
          }
        }
        n241 = Bundle By Name(cluster=w383, "User Added Targets"=w381) -> (w382:T8)
      }
      frame "Configure Target" {
        # "Update network settings/configuration of the selected RT target"
        n242 = Unbundle By Name(w405) -> ("Targets Information"=w409:T10[], "Filtered Targets"=w412:i32[])
        n243 = Decimal String To Number(string=w413) -> (number=w411:i32)  [unwired: 3 out]
        n244 = Index Array(array=w412, index=w411) -> (element=w407:i32)
        n245 = Index Array(array=w409, index=w407) -> (element=w410:T10)
        n246 = call "rad_Configure Target Dialog.vi"("Error In"=w399, "Target Information in"=w410) -> ("Error Out"=w400:errorcluster, "Target Information out"=w408:T10)  [unwired: 8 out]
        n247 = Replace Array Subset(array=w409, new element=w408, index=w407) -> (w406:T10[])
        n248 = call <vilib>:"General Error Handler.vi"("error in (no error)"=w400) -> ()  [unwired: 10 in, 5 out]
        n249 = Bundle By Name(cluster=w405, "Targets Information"=w406) -> (w404:T8)
        n250 = call "Enqueue Message with Data.vi"("error in (no error)"=w399, "message ID"="Update UI", "queue in"=w403) -> ("error out"=w401:errorcluster)  [unwired: 7 in, 1 out]
      }
      frame "Configure Targets Settings" {
        # "Update the RT Target settings >> select which types of RT targets to display in the table\nCompactRIO, PXI, FieldPoint, or Other"
        n251 = Unbundle By Name(w421) -> ("Targets Settings"=w416:T9)
        n252 = call "rad_Configure Targets Settings Dialog.vi"("Targets Settings"=w416) -> ("Targets Settings"=w417:T9)  [unwired: 10 out]
        n253 = Equal?(x=w417, y=w416) -> (x = y?=w414:bool)
        n254 = Bundle By Name(cluster=w421, "Targets Settings"=w417) -> (w420:T8)
        n255 = case shown="False" w414 {
          tunnel: w419 -> [w425 _]
          tunnel: w418 -> [w424 w426]
          tunnel: [w423 w426] -> w415
          frame False {
            n256 = call "Enqueue Message with Data.vi"("error in (no error)"=w424, "message ID"="Update UI", "queue in"=w425) -> ("error out"=w423:errorcluster)  [unwired: 7 in, 1 out]
          }
          frame True {
          }
        }
      }
      frame "View Target Info" {
        # "Display additional information about the selected RT target in a popup window"
        n257 = Unbundle By Name(w436) -> ("Targets Information"=w435:T10[], "Filtered Targets"=w433:i32[])
        n258 = Decimal String To Number(string=w434) -> (number=w432:i32)  [unwired: 3 out]
        n259 = Index Array(array=w433, index=w432) -> (element=w431:i32)
        n260 = Index Array(array=w435, index=w431) -> (element=w427:T10)
        n261 = call "rad_Get Target Info (IP).vi"("error in (no error)"=w429, "Target settings in"=w427) -> ("error out"=w428:errorcluster, "Target settings out"=w430:T10)  [unwired: 8 in]
        n262 = case shown="No Error" w428 {
          selector: w428 -> [_ w438]
          tunnel: w430 -> [w437 _]
          frame No Error {
            n263 = call "rad_Target Info Dialog.vi"("Target Information"=w437) -> ()  [unwired: 11 out]
          }
          frame Error {
            n264 = call <vilib>:"General Error Handler.vi"("error in (no error)"=w438) -> ()  [unwired: 10 in, 5 out]
          }
        }
      }
      frame "Delete Target" {
        n265 = Unbundle By Name(w454) -> ("Targets Information"=w453:T10[], "Filtered Targets"=w441:i32[], "User Added Targets"=w442:string[])
        n266 = Decimal String To Number(string=w458) -> (number=w444:i32)  [unwired: 2 in, 1 out]
        n267 = Index Array(array=w441, index=w444) -> (element=w443:i32)
        n268 = Delete From Array(array=w453, length=1, index=w443) -> (deleted portion=w451:T10[], array with subset deleted=w452:T10[])
        n269 = Index Array(array=w451) -> (element=w450:T10)  [unwired: 1 in]
        n270 = Unbundle By Name(w450) -> ("Primary NIC.IP address"=w440:string)
        n271 = Search 1D Array(1D array=w442, element=w440) -> (index of element=w457:i32)  [unwired: 1 in]
        n272 = call "Enqueue Message with Data.vi"("error in (no error)"=w447, "message ID"="Update UI" ("Message Name"), "queue in"=w448) -> ("error out"=w446:errorcluster)  [unwired: 7 in, 1 out]
        n273 = Delete From Array(array=w442, length=1, index=w457) -> (array with subset deleted=w439:string[])  [unwired: 1 out]
        n274 = Bundle By Name(cluster=w454, "Targets Information"=w452, "User Added Targets"=w439) -> (w449:T8)
      }
      frame "**** Image Messages ****" {
      }
      frame "Refresh AppImages" {
        # "Update list of application images available in the configured folder"
        n275 = Unbundle By Name(w466) -> ("App Images Settings.App Images Temp Folder"=w467:path, "App Images Settings.App Images Folder"=w471:path)
        n276 = call "Util_Progress Show Progress Popup.vi"("Title"="Refreshing App Images", "Message"="Refreshing application images list...") -> ("error out"=w470:errorcluster)  [unwired: 2 in, 7 out]
        n277 = call "rad_List Application Images.vi"("App Image Temp Folder"=w467, "error in (no error)"=w470, "App Images Folder"=w471) -> ("error out"=w469:errorcluster, "Application Images Infomration"=w468:T13[])  [unwired: 1 in, 6 out]
        n278 = Bundle By Name(cluster=w466, "App Images Information"=w468) -> (w462:T8)
        n279 = call "Util_Progress Close Progress Popup.vi"("error in (no error)"=w469) -> ()  [unwired: 2 in, 9 out]
        n280 = call "Enqueue Message with Data.vi"("error in (no error)"=w463, "message ID"="Update UI" ("Message"), "queue in"=w464) -> ("error out"=w465:errorcluster)  [unwired: 7 in, 1 out]
      }
      frame "Configure App Image" {
        # "Update additional information (name, verison, description)\nstored with the selected application image"
        n281 = Unbundle By Name(w484) -> ("App Images Settings.App Images Temp Folder"=w480:path, "App Images Information"=w486:T13[])
        n282 = Decimal String To Number(string=w487) -> (number=w482:i32)  [unwired: 3 out]
        n283 = Index Array(array=w486, index=w482) -> (element=w481:T13)
        n284 = call "rad_Configure Application Image.vi"("Temp Folder"=w480, "error in (no error)"=w479, "App Images Information"=w481) -> ("error out"=w476:errorcluster, "Cancelled"=w474:bool, "App Images Information"=w475:T13)  [unwired: 6 in]
        n285 = Replace Array Subset(array=w486, new element=w475, index=w482) -> (w485:T13[])
        n286 = case shown="False" w474 {
          tunnel: [w491 w492] -> w478
          tunnel: w477 -> [w489 _]
          tunnel: w476 -> [w488 w492]
          frame False {
            n287 = call "Enqueue Message with Data.vi"("error in (no error)"=w488, "message ID"="Refresh AppImages", "queue in"=w489) -> ("error out"=w491:errorcluster)  [unwired: 7 in, 1 out]
          }
          frame True {
          }
        }
        n288 = Bundle By Name(cluster=w484, "App Images Information"=w485) -> (w483:T8)
      }
      frame "Configure AppImages Settings" {
        # "Update the selection of the folder where application images are stored"
        n289 = Unbundle By Name(w497) -> ("App Images Settings"=w496:T12)
        n290 = call "rad_Configure App Images Settings Dialog.vi"("App Images Settings"=w496) -> ("Cancelled"=w493:bool, "App Images Settings"=w495:T12)  [unwired: 1 in, 8 out]
        n291 = case shown="False" w493 {
          tunnel: w500 -> [w504 _]
          tunnel: w499 -> [w502 w505]
          tunnel: [w501 w505] -> w494
          frame False {
            n292 = call "Enqueue Message with Data.vi"("error in (no error)"=w502, "message ID"="Refresh AppImages", "queue in"=w504) -> ("error out"=w501:errorcluster)  [unwired: 7 in, 1 out]
          }
          frame True {
          }
        }
        n293 = Bundle By Name(cluster=w497, "App Images Settings"=w495) -> (w498:T8)
      }
      frame "View App Image Info" {
        n294 = Unbundle By Name(w510) -> ("App Images Information"=w509:T13[])
        n295 = Decimal String To Number(string=w507) -> (number=w506:i32)  [unwired: 2 in, 1 out]
        n296 = Index Array(array=w509, index=w506) -> (element=w508:T13)
        n297 = call "rad_View App Image Info.vi"("App Images Information"=w508) -> ()  [unwired: 11 in]
      }
      frame "Compare App Image" {
        n298 = Scan From String(format string="%[^(]", input string=w514) -> (remaining string=w513:string, output 1=w515:string)  [unwired: 2 in, 3 out]
        n299 = case shown="\"Image Target Compare\"" w515 {
          tunnel: w518 -> [w530 w559 w565]
          tunnel: w517 -> [w527 w551 w570]
          tunnel: w513 -> [w529 w561 _]
          tunnel: [w522 w549 w569] -> w512
          frame "Image Target Compare" {
            n300 = Unbundle By Name(w530) -> ("App Images Settings.App Images Folder"=w521:path, "App Images Settings.App Images Temp Folder"=w525:path, "App Images Information"=w535:T13[], "Targets Information"=w531:T10[], "Filtered Targets"=w532:i32[])
            n301 = Scan From String(format string="(%[^)]):%d", input string=w529, error in=w527) -> (error out=w523:errorcluster, output 1=w534:string, output 2=w536:i32)  [unwired: 1 in, 4 out]
            n302 = while {
              shift-right: [w544] -> _
              shift-left: w534 -> [w546]
              tunnel: w532 -> [w541]
              tunnel: w531 -> [w539]
              tunnel: [w538] -> w528 mode=indexing
              stop <- w543 stop-if-true
              n303 = Scan From String(format string="%d,", input string=w546) -> (remaining string=w544:string, output 1=w540:i32)  [unwired: 2 in, 3 out]
              n304 = Index Array(array=w541, index=w540) -> (element=w542:i32)
              n305 = Empty String/Path?(string/path=w544) -> (empty?=w543:bool)
              n306 = Index Array(array=w539, index=w542) -> (element=w538:T10)
            }
            n307 = Index Array(array=w535, index=w536) -> (element=w533:T13)
            n308 = Index Array(array=w528) -> (element=w519:T10)  [unwired: 1 in]
            n309 = Unbundle By Name(w533) -> ("AppImage Path"=w526:path)
            n310 = call "rad_RT Image Compare Dialog.vi"("App Images Repository"=w521, "Begin Automatically? (F)"=TRUE ("Show Front Panel?"), "Temp Folder"=w525, "error in (no error)"=w523, "Operation"=rad_Comparison_Modes."Compare Local Image With Controller", "Target settings"=w519, "Original Image Path"=w526) -> ("error out"=w522:errorcluster)  [unwired: 4 in]
          }
          frame "Only Image Selected" {
            n311 = Unbundle By Name(w559) -> ("App Images Settings.App Images Folder"=w548:path, "App Images Settings.App Images Temp Folder"=w554:path, "App Images Information"=w558:T13[])
            n312 = Scan From String(format string="(%d", input string=w561, error in=w551) -> (error out=w550:errorcluster, output 1=w557:i32)  [unwired: 1 in, 3 out]
            n313 = Index Array(array=w558, index=w557) -> (element=w556:T13)
            n314 = Unbundle By Name(w556) -> ("AppImage Path"=w555:path)
            n315 = call "rad_RT Image Compare Dialog.vi"("App Images Repository"=w548, "Begin Automatically? (F)"=FALSE ("Operate Headlessly?"), "Temp Folder"=w554, "error in (no error)"=w550, "Operation"=rad_Comparison_Modes."Compare Local Image With Controller", "Target settings"=T10 {"Hostname"="", "Serial number"="", "Product name"="", "Product code"=0, "System status"="", "Credential type"=enum."None/Unlocked", "User added?"=FALSE, "Primary NIC"={"MAC address"="", "IP Address Request Mode"=0, "IP address"="", "Subnet mask"="", "Gateway"="", "DNS server"=""}}, "Original Image Path"=w555) -> ("error out"=w549:errorcluster)  [unwired: 4 in]
          }
          frame "Generic Compare", Default {
            n316 = Unbundle By Name(w565) -> ("App Images Settings.App Images Folder"=w563:path, "App Images Settings.App Images Temp Folder"=w564:path)
            n317 = call "rad_RT Image Compare Dialog.vi"("App Images Repository"=w563, "Begin Automatically? (F)"=FALSE ("Operate Headlessly?"), "Temp Folder"=w564, "error in (no error)"=w570, "Operation"=rad_Comparison_Modes."Compare Local Image With Controller", "Target settings"=T10 {"Hostname"="", "Serial number"="", "Product name"="", "Product code"=0, "System status"="", "Credential type"=enum."None/Unlocked", "User added?"=FALSE, "Primary NIC"={"MAC address"="", "IP Address Request Mode"=0, "IP address"="", "Subnet mask"="", "Gateway"="", "DNS server"=""}}, "Original Image Path"=path "") -> ("error out"=w569:errorcluster)  [unwired: 4 in]
          }
        }
      }
      frame "Delete App Image" {
        n318 = Unbundle By Name(w587) -> ("App Images Information"=w586:T13[])
        n319 = Decimal String To Number(string=w585) -> (number=w584:i32)  [unwired: 2 in, 1 out]
        n320 = Index Array(array=w586, index=w584) -> (element=w583:T13)
        n321 = Unbundle By Name(w583) -> ("AppImage Path"=w578:path, "AppImage Properties.Name"=w580:string, "AppImage Properties.Version"=w571:string)
        n322 = Concatenate Strings("Are you sure you want to delete " ("string"), w580, " version " ("string"), w571, "?" ("string")) -> (w579:string)
        n323 = Two Button Dialog(message=w579, 2:"Delete" ("button name (\"OK\")")) -> (T button?=w577:bool)  [unwired: 1 in]
        n324 = case shown="True" w577 {
          tunnel: w578 -> [_ w594]
          tunnel: w576 -> [w588 w593]
          tunnel: [w588 w591] -> w575
          tunnel: w574 -> [_ w590]
          frame False {
          }
          frame True {
            n325 = Delete(path (use dialog)=w594, error in=w593) -> (error out=w592:errorcluster)  [unwired: 3 in, 2 out]
            n326 = call "Enqueue Message with Data.vi"("error in (no error)"=w592, "message ID"="Refresh AppImages" ("Message Name"), "queue in"=w590) -> ("error out"=w591:errorcluster)  [unwired: 7 in, 1 out]
          }
        }
      }
      frame "Retrieve AppImage" {
        # "Retrieve the application image\nfrom the selected RT target."
        n327 = Unbundle By Name(w603) -> ("App Images Settings.App Images Temp Folder"=w605:path, "App Images Settings.App Images Folder"=w599:path, "Targets Information"=w595:T10[], "Filtered Targets"=w596:i32[])
        n328 = Decimal String To Number(string=w611) -> (number=w610:i32)  [unwired: 3 out]
        n329 = Index Array(array=w596, index=w610) -> (element=w612:i32)
        n330 = Index Array(array=w595, index=w612) -> (element=w597:T10)
        n331 = call "rad_Retrieve Application Image From Target.vi"("App Images Temp Folder"=w605, "error in (no error)"=w609, "Target settings"=w597, "App Images Folder"=w599) -> ("error out"=w608:errorcluster, "Cancelled"=w600:bool, "New App Image Path"=w604:path)  [unwired: 3 in, 2 out]
        n332 = Strip Path(path=w604) -> (stripped path=w601:path)  [unwired: 1 out]
        n333 = case shown="False" w600 {
          tunnel: w608 -> [w616 w617]
          tunnel: [w615 w617] -> w607
          tunnel: w606 -> [w614 _]
          frame False {
            n334 = call "Enqueue Message with Data.vi"("error in (no error)"=w616, "message ID"="Refresh AppImages" ("Message Name"), "queue in"=w614) -> ("error out"=w615:errorcluster)  [unwired: 7 in, 1 out]
          }
          frame True {
          }
        }
        n335 = Select(t=w599, s=w600, f=w601) -> (s? t:f=w598:path)
        n336 = Bundle By Name(cluster=w603, "App Images Settings.App Images Folder"=w598) -> (w602:T8)
      }
      frame "Deploy AppImage" {
        # "Deploy the selected application image to the select RT target(s)"
        n337 = Unbundle By Name(w634) -> ("App Images Settings.App Images Temp Folder"=w624:path, "App Images Information"=w630:T13[], "Targets Information"=w626:T10[], "Filtered Targets"=w627:i32[])
        n338 = Scan From String(format string="(%[^)]):%d", input string=w633) -> (output 1=w629:string, output 2=w631:i32)  [unwired: 2 in, 5 out]
        n339 = while {
          shift-right: [w646] -> _
          shift-left: w629 -> [w648]
          tunnel: w627 -> [w643]
          tunnel: w626 -> [w641]
          tunnel: [w640] -> w623 mode=indexing
          stop <- w645 stop-if-true
          n340 = Scan From String(format string="%d,", input string=w648) -> (remaining string=w646:string, output 1=w642:i32)  [unwired: 2 in, 3 out]
          n341 = Index Array(array=w643, index=w642) -> (element=w644:i32)
          n342 = Empty String/Path?(string/path=w646) -> (empty?=w645:bool)
          n343 = Index Array(array=w641, index=w644) -> (element=w640:T10)
        }
        n344 = Index Array(array=w630, index=w631) -> (element=w628:T13)
        n345 = Unbundle By Name(w628) -> ("AppImage Path"=w625:path)
        n346 = call "rad_Deploy Application Image.vi"("App Image Temp Folder"=w624, "error in (no error)"=w622, "Selected Targets"=w623, "App Image Path"=w625) -> ("error out"=w620:errorcluster, "Cancelled"=w618:bool)  [unwired: 6 out]
        n347 = case shown="False" w618 {
          tunnel: [w638 w639] -> w621
          tunnel: w620 -> [w637 w639]
          tunnel: w619 -> [w635 _]
          frame False {
            n348 = call "Enqueue Message with Data.vi"("error in (no error)"=w637, "message ID"="Refresh Targets" ("Message Name"), "queue in"=w635) -> ("error out"=w638:errorcluster)  [unwired: 7 in, 1 out]
          }
          frame True {
          }
        }
      }
      frame "Convert Images" {
        n349 = Unbundle By Name(w650) -> ("App Images Settings.App Images Folder"=w649:path)
        n350 = call "Util_ConvertImageToLatest.vi"("error in (no error)"=w655, "Image Path"=w649) -> ("error out"=w653:errorcluster)  [unwired: 9 in]
        n351 = call "Enqueue Message with Data.vi"("error in (no error)"=w653, "message ID"="Refresh AppImages" ("Message Name"), "queue in"=w651) -> ("error out"=w652:errorcluster)  [unwired: 7 in, 1 out]
      }
    }
    n352 = local write "State"(w171) -> ()
  }
  n353 = call "Resize Front Panel Main.vi"("Left Listbox"=w29, "Top Level VI"=w30, "Stop"=w31, "Number of Columns"=4, "Right Listbox"=w28, "Left Splitter"=w27, "Right Splitter"=w26, "Left Pane Items"=w20, "Mid Pane Items"=w16, "Right Pane Items"=w11) -> ()  [unwired: 5 in, 1 out]
  n354 = local write "Exit"(w10) -> ()
